vi "SetADChannels.vi"(0 "error out":errorcluster, 1 "Numeric":i32, 2 "Boolean":bool) -> (3 "error out 2":errorcluster, 6 "Numeric 2":i32)   [LabVIEW 2009]
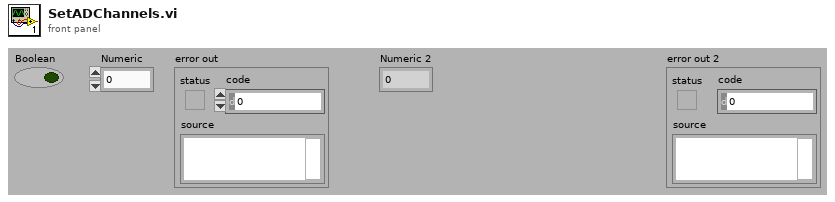
[diagram p1: front panel]
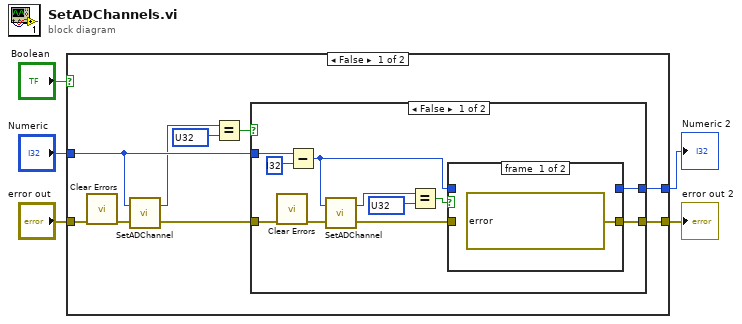
[diagram p0: block diagram]
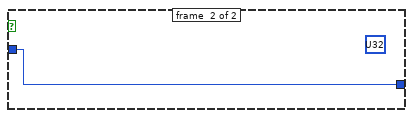
[diagram p3: hidden frame]
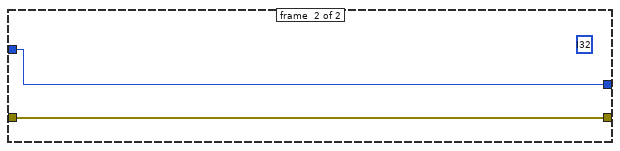
[diagram p4: hidden frame]
diagram:
  n1 = case shown="False" "Boolean" {
    tunnel: "error out" -> [w14 w30]
    tunnel: [w9 w30] -> w1
    tunnel: [w8 w31] -> w2
    tunnel: "Numeric" -> [w7 w31]
    frame #0 {
      n2 = call <vilib>:"Clear Errors.vi"("error in (no error)"=w14) -> ("error out"=w12:errorcluster)  [unwired: 6 in]
      n3 = call "SetADChannel.vi"("error in (no error)"=w12, "channel"=w7) -> ("error out"=w10:errorcluster, "DLL error code"=w6:u32)
      n4 = Equal?(x=w6, y=u32 ?) -> (x = y?=w11:bool)
      n5 = case shown="False" w11 {
        tunnel: w10 -> [w19 _]
        tunnel: w7 -> [w25 w29]
        tunnel: [w20 _] -> w9
        tunnel: [w16 w29] -> w8
        frame #0 {
          n6 = call <vilib>:"Clear Errors.vi"("error in (no error)"=w19) -> ("error out"=w18:errorcluster)  [unwired: 6 in]
          n7 = Subtract(x=w25, y=i32 ?) -> (x-y=w17:i32)
          n8 = call "SetADChannel.vi"("error in (no error)"=w18, "channel"=w17) -> ("error out"=w21:errorcluster, "DLL error code"=w15:u32)
          n9 = Equal?(x=w15, y=u32 ?) -> (x = y?=w22:bool)
          n10 = case shown="True" w22 {
            tunnel: [errorcluster ? ("error out") w28] -> w20
            tunnel: w21 -> [_ w28]
            tunnel: w17 -> [_ w27]
            tunnel: [_ w27] -> w16
            frame #0 {
            }
            frame #1 {
            }
          }
        }
        frame #1 {
          (unwired) u32 ? ("DLL error code")
        }
      }
    }
    frame #1 {
      (unwired) i32 ?
    }
  }
  "Numeric 2" <- w2
  "error out 2" <- w1
